vi "dequeueElem.vi"(8 "error_in":errorcluster, 11 "queue_in":refnum<queue>) -> (0 "error_out":errorcluster, 2 "element_out":T1, 3 "queue_out":refnum<queue>)   [LabVIEW 2017]
uses:
  controls/stateMachine.ctl
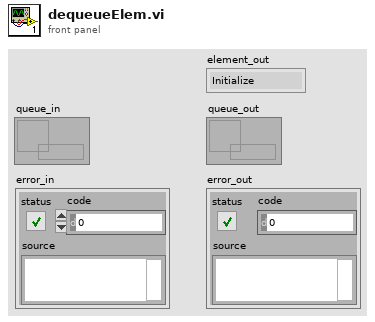
[diagram p1: front panel]
types:
  T1 = typedef "stateMachine.ctl" = enum16{"Initialize", "Start", "Pause", "Stop", "Shutdown"}
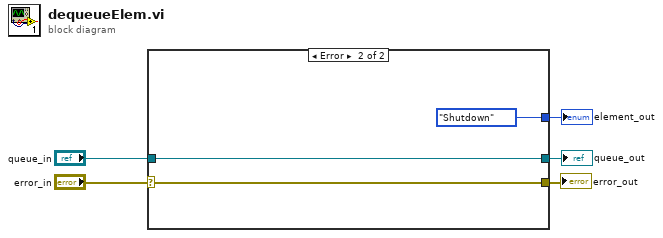
[diagram p0: block diagram]
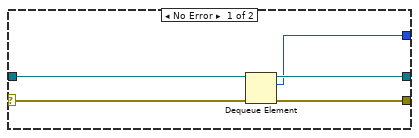
[diagram p2: hidden frame]
diagram:
  n1 = case shown="Error" "error_in" {
    selector: "error_in" -> [w10 w13]
    tunnel: [w9 w13] -> w2
    tunnel: [w8 w12] -> w3
    tunnel: "queue_in" -> [w7 w12]
    tunnel: [w6 stateMachine."Shutdown" ("element")] -> w1
    frame No Error {
      n2 = Dequeue Element(queue=w7, error in (no error)=w10) -> (queue out=w8:refnum<queue>, element=w6:T1, error out=w9:errorcluster)  [unwired: 1 in, 1 out]
    }
    frame Error {
    }
  }
  "queue_out" <- w3
  "error_out" <- w2
  "element_out" <- w1
